vi "Autotuning Help.vi"() -> ()   [LabVIEW 2017, in "NI_PID_autopid.lvlib"]
uses:
  <vilib>/addons/control/pid/NI_PID_autopid.lvlib
  <vilib>/addons/control/pid/_autopid compat.llb/State.gbl.vi
  <vilib>/addons/control/pid/NI_PID__autopid compat.lvlib
panel:
  in  "?":bool
  in  "Instructions":string
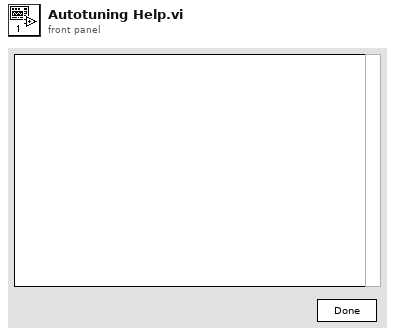
[diagram p1: front panel]
types:
  T1 = enum16{"Normal", "Start", "Check params", "Check noise", "Start noise est.", "Re-estimate noise", "Begin autotune", "Autotuning", "New parameters", ""}
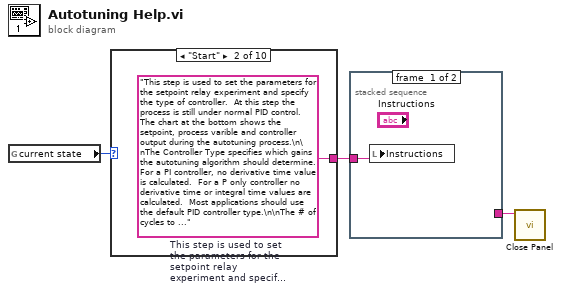
[diagram p0: block diagram]
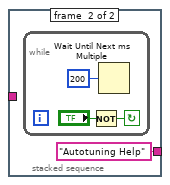
[diagram p2: hidden frame]
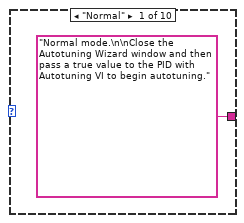
[diagram p3: hidden frame]
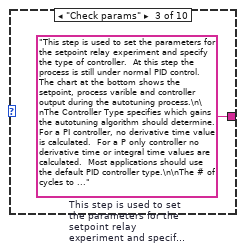
[diagram p4: hidden frame]
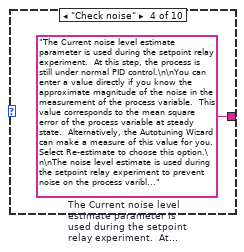
[diagram p5: hidden frame]
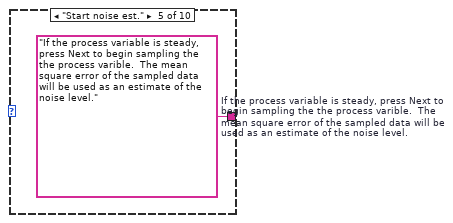
[diagram p6: hidden frame]
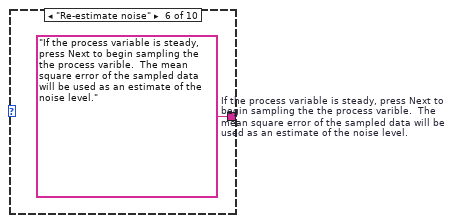
[diagram p7: hidden frame]
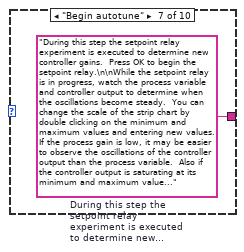
[diagram p8: hidden frame]
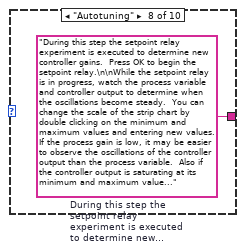
[diagram p9: hidden frame]
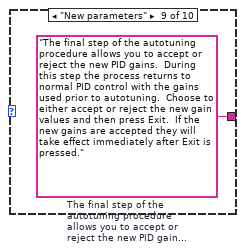
[diagram p10: hidden frame]
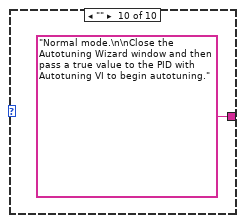
[diagram p11: hidden frame]
diagram:
  n1 = global read "State.gbl.vi" "current state"() -> (w3:T1)
  n2 = case shown="\"Start\"" w3 {
    tunnel: ["Normal mode.\n\nClose the Autotuning Wizard window and then pass a true value to the PID with Autotuning VI to begin autotuning." w5 w6 w7 w8 w9 w10 w11 w12 "Normal mode.\n\nClose the Autotuning Wizard window and then pass a true value to the PID with Autotuning VI to begin autotuning."] -> w2
    frame "Normal" {
    }
    frame "Start" {
      w5 = "This step is used to set the parameters for the setpoint relay experiment and specify the type of controller.  At this step the process is still under normal PID control.  The chart at the bottom shows the setpoint, process varible and controller output during the autotuning process.\n\nThe Controller Type specifies which gains the autotuning algorithm should determine.  For a PI controller, no derivative time value is calculated.  For a P only controller no derivative time or integral time values are calculated.  Most applications should use the default PID controller type.\n\nThe # of cycles to avg is used during the setpoint relay experiment.  When the setpoint relay oscillations are steady, the autotuning algorithm uses # of cycles to avg cycles to determine the average period and amplitude of the oscillations.  More cycles averaged will produce better results, but for some slow processes you may want to reduce this number to speed up the autotuning process.\n\nRelay amplitude is also used during the setpoint relay experiment.  This parameter specifies the step change of the current setpoint up and down.  For example, if setpoint is 40 and Relay amplitude is 2, the setpoint relay experiment will cycle the setpoint between 38 and 42.\n\nThe selection of the Relay amplitude parameter is very important for the autotuning process.  Ideally this value should be set large enough such that during the setpoint relay experiment each oscillation period takes at least 20 control cycles.  However, note that the autotuning algorithm assumes a linear plant model and controller.  If the Relay amplitude is set too high, the controller output will saturate at its maximum and minimum values during setpoint relay and the results will be invalid.  In this case, lower the Relay amplitude value and begin the autotuning procedure again.\n\nThe Control design parameter specifies the preferred performance of the tuned PID gains.  Normal parameters will generally yield fast response with minimal overshoot.  Fast performance will normally have a faster rise time but some overshoot of the setpoint.  Slow performance will be overdamped and will typically not have overshoot."  # This step is used to set the parameters for the setpoint relay experiment and specify the type of controller.  At this step the process is still under normal PID control.  The chart at the bottom shows the setpoint, process varible and controller output during the autotuning process.  The Controller Type specifies which gains the autotuning algorithm should determine.  For a PI controller, no derivative time value is calculated.  For a P only controller no derivative time or integral time values are calculated.  Most applications should use the default PID controller type.  The # of cycles to avg is used during the setpoint relay experiment.  When the setpoint relay oscillations are steady, the autotuning algorithm uses # of cycles to avg cycles to determine the average period and amplitude of the oscillations.  More cycles averaged will produce better results, but for some slow processes you may want to reduce this number to speed up the autotuning process.  Relay amplitude is also used during the setpoint relay experiment.  This parameter specifies the step change of the current setpoint up and down.  For example, if setpoint is 40 and Relay amplitude is 2, the setpoint relay experiment will cycle the setpoint between 38 and 42.  The selection of the Relay amplitude parameter is very important for the autotuning process.  Ideally this value should be set large enough such that during the setpoint relay experiment each oscillation period takes at least 20 control cycles.  However, note that the autotuning algorithm assumes a linear plant model and controller.  If the Relay amplitude is set too high, the controller output will saturate at its maximum and minimum values during setpoint relay and the results will be invalid.  In this case, lower the Relay amplitude value and begin the autotuning procedure again.  The Control design parameter specifies the preferred performance of the tuned PID gains.  Normal parameters will generally yield fast response with minimal overshoot.  Fast performance will normally have a faster rise time but some overshoot of the setpoint.  Slow performance will be overdamped and will typically not have overshoot.
    }
    frame "Check params" {
      w6 = "This step is used to set the parameters for the setpoint relay experiment and specify the type of controller.  At this step the process is still under normal PID control.  The chart at the bottom shows the setpoint, process varible and controller output during the autotuning process.\n\nThe Controller Type specifies which gains the autotuning algorithm should determine.  For a PI controller, no derivative time value is calculated.  For a P only controller no derivative time or integral time values are calculated.  Most applications should use the default PID controller type.\n\nThe # of cycles to avg is used during the setpoint relay experiment.  When the setpoint relay oscillations are steady, the autotuning algorithm uses # of cycles to avg cycles to determine the average period and amplitude of the oscillations.  More cycles averaged will produce better results, but for some slow processes you may want to reduce this number to speed up the autotuning process.\n\nRelay amplitude is also used during the setpoint relay experiment.  This parameter specifies the step change of the current setpoint up and down.  For example, if setpoint is 40 and Relay amplitude is 2, the setpoint relay experiment will cycle the setpoint between 38 and 42.\n\nThe selection of the Relay amplitude parameter is very important for the autotuning process.  Ideally this value should be set large enough such that during the setpoint relay experiment each oscillation period takes at least 20 control cycles.  However, note that the autotuning algorithm assumes a linear plant model and controller.  If the Relay amplitude is set too high, the controller output will saturate at its maximum and minimum values during setpoint relay and the results will be invalid.  In this case, lower the Relay amplitude value and begin the autotuning procedure again.\n\nThe Control design parameter specifies the preferred performance of the tuned PID gains.  Normal parameters will generally yield fast response with minimal overshoot.  Fast performance will normally have a faster rise time but some overshoot of the setpoint.  Slow performance will be overdamped and will typically not have overshoot."  # This step is used to set the parameters for the setpoint relay experiment and specify the type of controller.  At this step the process is still under normal PID control.  The chart at the bottom shows the setpoint, process varible and controller output during the autotuning process.  The Controller Type specifies which gains the autotuning algorithm should determine.  For a PI controller, no derivative time value is calculated.  For a P only controller no derivative time or integral time values are calculated.  Most applications should use the default PID controller type.  The # of cycles to avg is used during the setpoint relay experiment.  When the setpoint relay oscillations are steady, the autotuning algorithm uses # of cycles to avg cycles to determine the average period and amplitude of the oscillations.  More cycles averaged will produce better results, but for some slow processes you may want to reduce this number to speed up the autotuning process.  Relay amplitude is also used during the setpoint relay experiment.  This parameter specifies the step change of the current setpoint up and down.  For example, if setpoint is 40 and Relay amplitude is 2, the setpoint relay experiment will cycle the setpoint between 38 and 42.  The selection of the Relay amplitude parameter is very important for the autotuning process.  Ideally this value should be set large enough such that during the setpoint relay experiment each oscillation period takes at least 20 control cycles.  However, note that the autotuning algorithm assumes a linear plant model and controller.  If the Relay amplitude is set too high, the controller output will saturate at its maximum and minimum values during setpoint relay and the results will be invalid.  In this case, lower the Relay amplitude value and begin the autotuning procedure again.  The Control design parameter specifies the preferred performance of the tuned PID gains.  Normal parameters will generally yield fast response with minimal overshoot.  Fast performance will normally have a faster rise time but some overshoot of the setpoint.  Slow performance will be overdamped and will typically not have overshoot.
    }
    frame "Check noise" {
      w7 = "The Current noise level estimate parameter is used during the setpoint relay experiment.  At this step, the process is still under normal PID control.\n\nYou can enter a value directly if you know the approximate magnitude of the noise in the measurement of the process variable.  This value corresponds to the mean square error of the process variable at steady state.  Alternatively, the Autotuning Wizard can make a measure of this value for you.  Select Re-estimate to choose this option.\n\nThe noise level estimate is used during the setpoint relay experiment to prevent noise on the process varible from triggering the relay.  The autotuning algorithm uses this noise level estimate as a hysterisis for the relay action."  # The Current noise level estimate parameter is used during the setpoint relay experiment.  At this step, the process is still under normal PID control.  You can enter a value directly if you know the approximate magnitude of the noise in the measurement of the process variable.  This value corresponds to the mean square error of the process variable at steady state.  Alternatively, the Autotuning Wizard can make a measure of this value for you.  Select Re-estimate to choose this option.  The noise level estimate is used during the setpoint relay experiment to prevent noise on the process varible from triggering the relay.  The autotuning algorithm uses this noise level estimate as a hysterisis for the relay action.
    }
    frame "Start noise est." {
      w8 = "If the process variable is steady, press Next to begin sampling the the process varible.  The mean square error of the sampled data will be used as an estimate of the noise level."  # If the process variable is steady, press Next to begin sampling the the process varible.  The mean square error of the sampled data will be used as an estimate of the noise level.
    }
    frame "Re-estimate noise" {
      w9 = "If the process variable is steady, press Next to begin sampling the the process varible.  The mean square error of the sampled data will be used as an estimate of the noise level."  # If the process variable is steady, press Next to begin sampling the the process varible.  The mean square error of the sampled data will be used as an estimate of the noise level.
    }
    frame "Begin autotune" {
      w10 = "During this step the setpoint relay experiment is executed to determine new controller gains.  Press OK to begin the setpoint relay.\n\nWhile the setpoint relay is in progress, watch the process variable and controller output to determine when the oscillations become steady.  You can change the scale of the strip chart by double clicking on the minimum and maximum values and entering new values.  If the process gain is low, it may be easier to observe the oscillations of the controller output than the process variable.  Also if the controller output is saturating at its minimum and maximum values you should restart the autotuning process and select a lower Relay amplitude.\n\nWhen the oscillations are steady press OK again.  After the specified number of relay cycles have elapsed the autotuning process will be complete.\n\n"  # During this step the setpoint relay experiment is executed to determine new controller gains.  Press OK to begin the setpoint relay.  While the setpoint relay is in progress, watch the process variable and controller output to determine when the oscillations become steady.  You can change the scale of the strip chart by double clicking on the minimum and maximum values and entering new values.  If the process gain is low, it may be easier to observe the oscillations of the controller output than the process variable.  Also if the controller output is saturating at its minimum and maximum values you should restart the autotuning process and select a lower Relay amplitude.  When the oscillations are steady press OK again.  After the specified number of relay cycles have elapsed the autotuning process will be complete.
    }
    frame "Autotuning" {
      w11 = "During this step the setpoint relay experiment is executed to determine new controller gains.  Press OK to begin the setpoint relay.\n\nWhile the setpoint relay is in progress, watch the process variable and controller output to determine when the oscillations become steady.  You can change the scale of the strip chart by double clicking on the minimum and maximum values and entering new values.  If the process gain is low, it may be easier to observe the oscillations of the controller output than the process variable.  Also if the controller output is saturating at its minimum and maximum values you should restart the autotuning process and select a lower Relay amplitude.\n\nWhen the oscillations are steady press OK again.  After the specified number of relay cycles have elapsed the autotuning process will be complete.\n\n"  # During this step the setpoint relay experiment is executed to determine new controller gains.  Press OK to begin the setpoint relay.  While the setpoint relay is in progress, watch the process variable and controller output to determine when the oscillations become steady.  You can change the scale of the strip chart by double clicking on the minimum and maximum values and entering new values.  If the process gain is low, it may be easier to observe the oscillations of the controller output than the process variable.  Also if the controller output is saturating at its minimum and maximum values you should restart the autotuning process and select a lower Relay amplitude.  When the oscillations are steady press OK again.  After the specified number of relay cycles have elapsed the autotuning process will be complete.
    }
    frame "New parameters" {
      w12 = "The final step of the autotuning procedure allows you to accept or reject the new PID gains.  During this step the process returns to normal PID control with the gains used prior to autotuning.  Choose to either accept or reject the new gain values and then press Exit.  If the new gains are accepted they will take effect immediately after Exit is pressed."  # The final step of the autotuning procedure allows you to accept or reject the new PID gains.  During this step the process returns to normal PID control with the gains used prior to autotuning.  Choose to either accept or reject the new gain values and then press Exit.  If the new gains are accepted they will take effect immediately after Exit is pressed.
    }
    frame "" {
    }
  }
  n3 = stacked-sequence {
    tunnel: w2 -> [w14 _]
    tunnel: [_ "Autotuning Help" ("VI name")] -> w1
    frame #0 {
      n4 = local write "Instructions"(w14) -> ()
    }
    frame #1 {
      n5 = while {
        stop <- w17 continue-if-true
        n6 = Not(x="?") -> (.not. x?=w17:bool)
        n7 = Wait Until Next ms Multiple(millisecond multiple=u32 200) -> ()  [unwired: 1 out]
      }
    }
  }
  n8 = call <vilib>:"Close Panel.vi"("VI name"=w1) -> ()  [unwired: 1 in, 10 out]
